vi "ModulatorUsage.vi"() -> ()   [LabVIEW 2017]
uses:
  FPGA/modInput.ctl
  FPGA/modOutput.ctl
  <vilib>/Platform/TimedLoop/XDataNode/timing_clust.ctl
  <vilib>/Platform/TimedLoop/XDataNode/nitl_modes.ctl
  <vilib>/Platform/TimedLoop/XDataNode/wakeup.ctl
  <vilib>/rvi/Emulation/niFpgaSctlEmulationGetInTimedLoop.vi
  <vilib>/rvi/Emulation/niFpgaEmulationReportErrorSimple.vi
  <vilib>/rvi/Emulation/niFpgaGetClockAttributes.vi
  <vilib>/rvi/Emulation/niFpgaCriticalErrorInLSC.vi
  <vilib>/Platform/TimedLoop/XDataNode/XDataNode.xnode
  <vilib>/Platform/TimedLoop/XDataNode/XDNodeRunTimeDep.lvlib
  FPGA/BuckBoost.lvlib
panel:
  out "output":T1[](array[typedef])
  in  "Enable":bool
  in  "input":T2={"signal"=[0.0, 0.0, 0.0, 0.0]}
  # "Device Utilization\n---------------------------\nTotal Slices: 21.3% (2832 out of 13300)\nSlice Registers: 8.0% (8493 out of 106400)\nSlice LUTs: 15.5% (8239 out of 53200)\nBlock RAMs: 3.6% (5 out of 140)\nDSP48s: 0.0% (0 out of 220)"
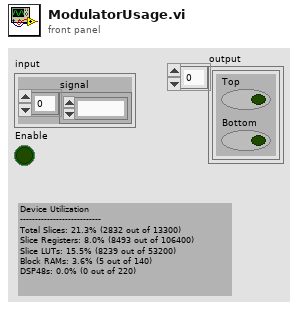
[diagram p1: front panel]
types:
  T1 = typedef "BuckBoost.lvlib/modOutput.ctl" = cluster{"Top":bool, "Bottom":bool}
  T2 = typedef "BuckBoost.lvlib/modInput.ctl" = cluster{"signal":fxp<+,18,0>[]}
  T3 = typedef "BuckBoost.lvlib/modRegisters.ctl" = cluster{"numberOfInterleaves":refnum<k21>, "Enable":refnum<k21>, "triangleInc":refnum<k21>, "Deadband":refnum<k21>}
  T4 = typedef "XDNodeRunTimeDep.lvlib/timing_clust.ctl" = cluster{"Expected End [f-1]":u64, "Actual End [f-1]":u64, "Finished Late? [f-1]":bool, "Expected End [i-1]":u64, "Actual End [i-1]":u64, "Finished Late? [i-1]":bool, "Expected Start [i]":u64, "Actual Start [i]":u64, "Expected Start [f]":u64, "Actual Start [f]":u64, "Source Name":string, "Structure Name":string, "Period":i64, "Deadline":i64, "Offset":i64, "Start":i64, "Priority":i32, "Timeout":i32, "Mode":T5, "Wakeup Reason":T6, "Error":errorcluster, "Source Type":string, "Secondary Source Type":string, "Global End Time":u64, "Global Start Time":u64, "Frame Duration":u64, "Iteration Duration":u64, "Assigned CPU":i32, "I/O Scan Engine Mode":u32}
  T5 = typedef "XDNodeRunTimeDep.lvlib/nitl_modes.ctl" = enum32{"No Change", "Process missed periods, maintain original phase", "Discard missed periods, maintain original phase", "Process missed periods, ignore original phase", "Discard missed periods, ignore original phase"}
  T6 = typedef "XDNodeRunTimeDep.lvlib/wakeup.ctl" = enum32{"Normal", "Aborted", "Asynchronous wakeup", "Timing source error", "Timed loop error", "Timeout"}
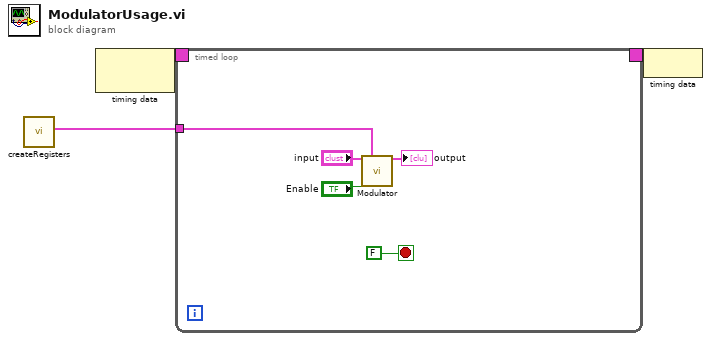
[diagram p0: block diagram]
diagram:
  n1 = call "createRegisters.vi"() -> ("modRegisters"=w1:T3)  [unwired: 10 in, 1 out]
  n2 = node-c288() -> (w3:T4)  [unwired: 1 in]
  n3 = timed-loop {
    timing: w3 -> [_]
    timing-out: [_] -> w2
    tunnel: w1 -> [w8]
    stop <- FALSE stop-if-true
    n4 = call "Modulator.vi"("input"="input", "modRegisters"=w8, "Disable"="Enable") -> ("output"=→"output":T1[])  [unwired: 12 in]
  }
  n5 = node-c288(w2) -> ()
